vi "HEWH FHD End Index.vi"(7 "Fixed Search?":bool, 8 "error in (no error)":errorcluster, 9 "Fixed Search Value":dbl format="%#_13g", 10 "RTDout":dbl[](array[numeric]), 11 "Draw Index":i32[](array[numeric])) -> (0 "error out":errorcluster, 2 "Decrement Amount":i32, 3 "Updated FHD End Index":i32[](array[numeric]))   [LabVIEW 2023]
panel:
  out "Reversed Array":dbl[](array[numeric])
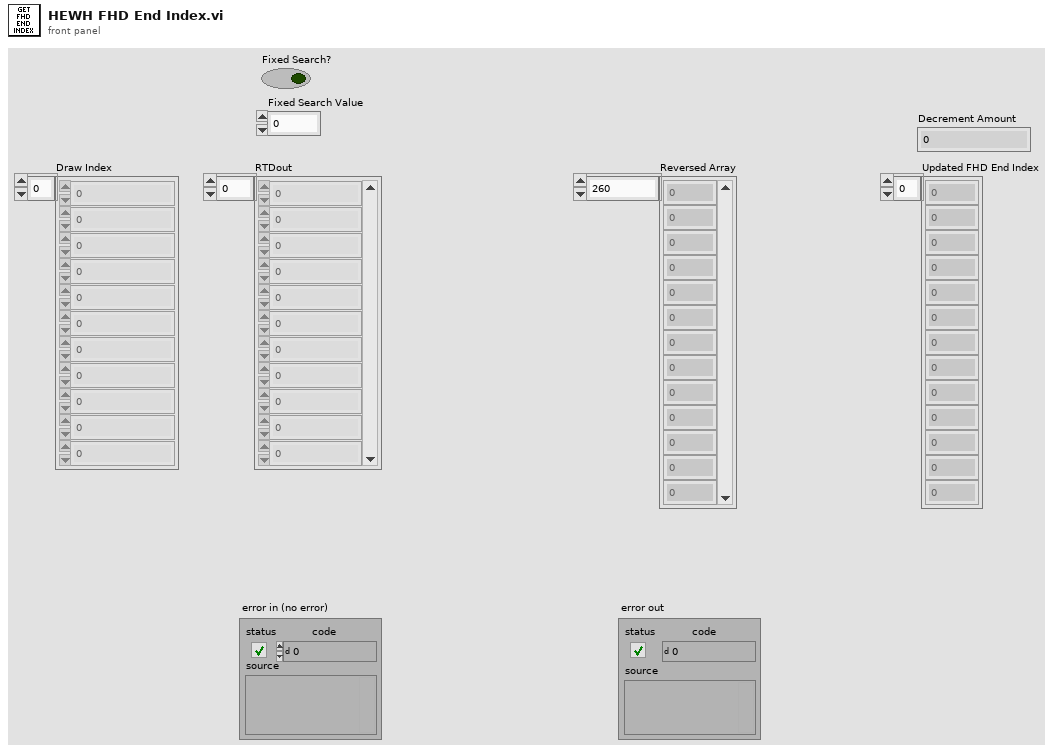
[diagram p1: front panel]
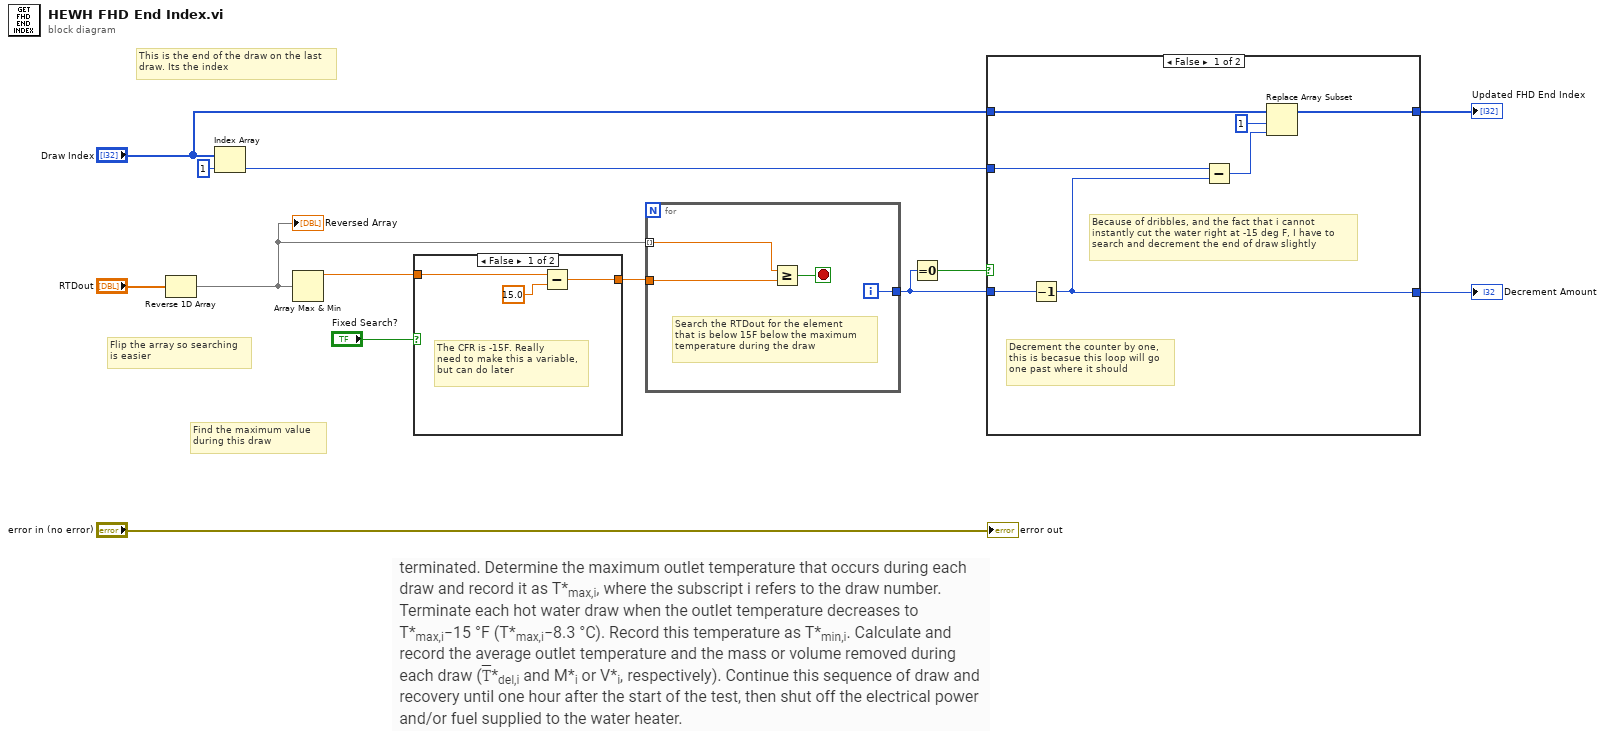
[diagram p0: block diagram]
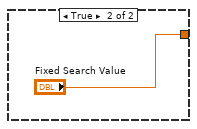
[diagram p2: hidden frame]
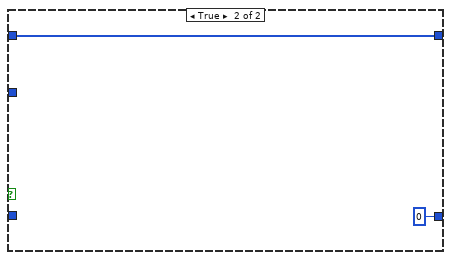
[diagram p3: hidden frame]
diagram:
  # "This is the end of the draw on the last\ndraw. Its the index"
  # "Flip the array so searching \nis easier"
  # "Find the maximum value\nduring this draw"
  n1 = Reverse 1D Array(array="RTDout") -> (reversed array=w4:dbl[])
  "Reversed Array" <- w4
  n2 = Index Array(array="Draw Index", index=1) -> (element=w8:i32)
  n3 = Array Max & Min(array=w4) -> (max value=w12:dbl)  [unwired: 3 out]
  n4 = case shown="False" "Fixed Search?" {
    tunnel: w12 -> [w15 _]
    tunnel: [w14 "Fixed Search Value"] -> w11
    frame False {
      # "The CFR is -15F. Really\nneed to make this a variable,\nbut can do later"
      n5 = Subtract(x=w15, y=15.0) -> (x-y=w14:dbl)
    }
    frame True {
    }
  }
  n6 = for {
    tunnel: w4 -> [w21] mode=indexing
    tunnel: [w19] -> w3
    tunnel: w11 -> [w18]
    i -> [w19]
    stop <- w20 stop-if-true
    # "Search the RTDout for the element\nthat is below 15F below the maximum\ntemperature during the draw"
    n7 = Greater Or Equal?(x=w21, y=w18) -> (x >= y?=w20:bool)
  }
  n8 = Equal To 0?(x=w3) -> (x = 0?=w2:bool)
  n9 = case shown="False" w2 {
    tunnel: w3 -> [w28 _]
    tunnel: [w27 0] -> w10
    tunnel: w8 -> [w26 _]
    tunnel: [w23 w30] -> w7
    tunnel: "Draw Index" -> [w22 w30]
    frame False {
      # "Decrement the counter by one,\nthis is becasue this loop will go\none past where it should"
      # "Because of dribbles, and the fact that i cannot\ninstantly cut the water right at -15 deg F, I have to \nsearch and decrement the end of draw slightly"
      n10 = Decrement(x=w28) -> (x-1=w27:i32)
      n11 = Subtract(x=w26, y=w27) -> (x-y=w24:i32)
      n12 = Replace Array Subset(array=w22, new element=w24, index=1) -> (w23:i32[])
    }
    frame True {
    }
  }
  "Updated FHD End Index" <- w7
  "Decrement Amount" <- w10
  "error out" <- "error in (no error)"
